vi "p11y1-2.vi"   [LabVIEW 2020]
uses:
  Global 1.vi
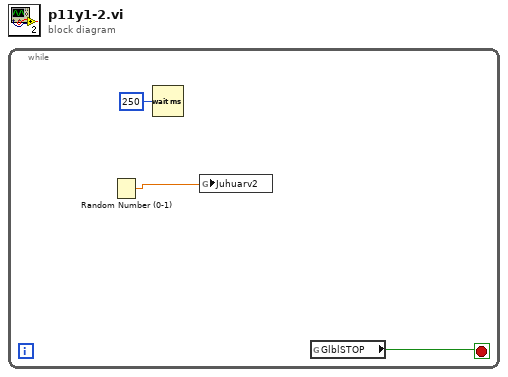
[diagram p0: block diagram]
diagram:
  n1 = while {
    stop <- w3 stop-if-true
    n2 = Random Number (0-1)() -> (number: 0 to 1=w1:dbl)
    n3 = Wait (ms)(milliseconds to wait=u32 250) -> ()  [unwired: 1 out]
    n4 = global write "Global 1.vi" "Juhuarv2"(w1) -> ()
    n5 = global read "Global 1.vi" "GlblSTOP"() -> (w3:bool)
  }
